vi "Variant to Class.vi"(8 "error in (no error)":errorcluster, 10 "Data in":variant, 11 "VIP Publish Node in":refnum<class "VIP Publish Node.lvclass">) -> (0 "error out":errorcluster, 2 "Data Out":variant, 3 "VIP Publish Node out":refnum<class "VIP Publish Node.lvclass">)   [LabVIEW 2014, in "VIP Publish Node.lvclass"]
uses:
  VIP Publish Node.lvclass
  Shared/Controls/VIP Publish - STYP.ctl
  VIP Publish Node.lvclass/VIP Publish Node.ctl
  Classes/Build Job/Build Job.lvclass
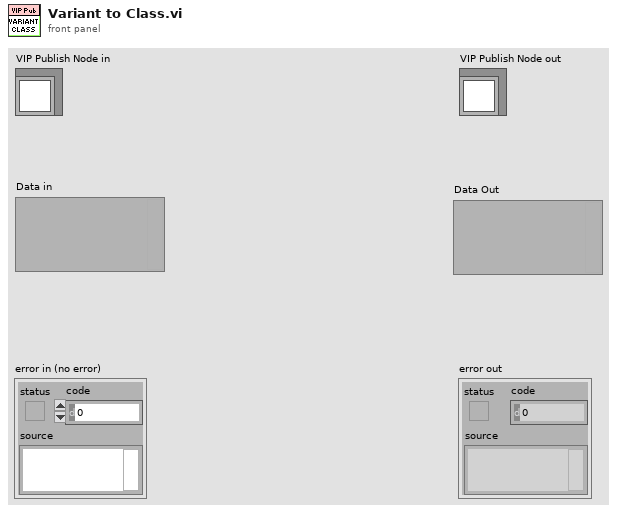
[diagram p1: front panel]
types:
  T1 = typedef "VIP Publish - STYP.ctl" = cluster{"VIP Path":string, "Repo Name":string}
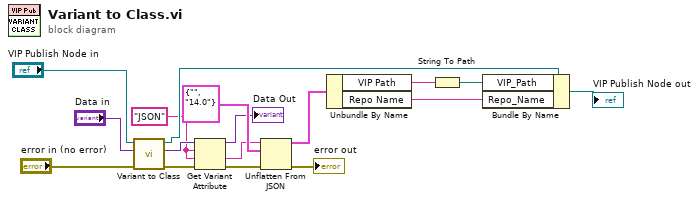
[diagram p0: block diagram]
diagram:
  w5 = "JSON" ("name")
  n1 = call-parent "Variant to Class.vi"("error in (no error)"="error in (no error)", "Data in"="Data in", "Build Job in"="VIP Publish Node in") -> ("error out"=w4:errorcluster, "Data Out"=w7:variant, "Build Job out"=w8:refnum<class "VIP Publish Node.lvclass">)  [unwired: 6 in]
  n2 = Get Variant Attribute(Variant=w7, name=w5, default value (empty Variant)=w5, error in=w4) -> (duplicate Variant=→"Data Out":variant, value=w10:string, error out=w9:errorcluster)  [unwired: 1 out]
  n3 = Unflatten From JSON(JSON string=w10, type and defaults=T1 {"VIP Path"="", "Repo Name"="14.0"} ("VIPB Build"), error in (no error)=w9) -> (value=w12:T1, error out=→"error out":errorcluster)  [unwired: 4 in]
  n4 = Unbundle By Name(w12) -> ("VIP Path"=w13:string, "Repo Name"=w1:string)
  n5 = String To Path(string=w13) -> (path=w14:path)
  n6 = Bundle By Name(cluster=w8, "VIP_Path"=w14, "Repo_Name"=w1) -> (→"VIP Publish Node out":refnum<class "VIP Publish Node.lvclass">)
